vi "LABVIEW_0416043.vi"() -> ()   [LabVIEW 2012]
uses:
  <vilib>/Utility/file.llb/Read From Spreadsheet File (DBL).vi
  <vilib>/Analysis/2dsp.llb/Real FFT.vi
  <vilib>/Analysis/NI_AALPro.lvlib
panel:
  out "Numeric 2":ext
  out "Numeric":ext
  out "FFT {X}":dbl[][](graph)
  out "CSV file path":path
  out "Input1":dbl[](graph)
  # "1. ¶}±ÒÀÉ®×¡AÆ[¹îŠ‹xe®t²§¡C  (ÀÉ¦W:XXX.csv)"
  # "4. HTþsŠ‹xe„vFFT"
  # "3. iQŠ‹xeKNBfßWW"
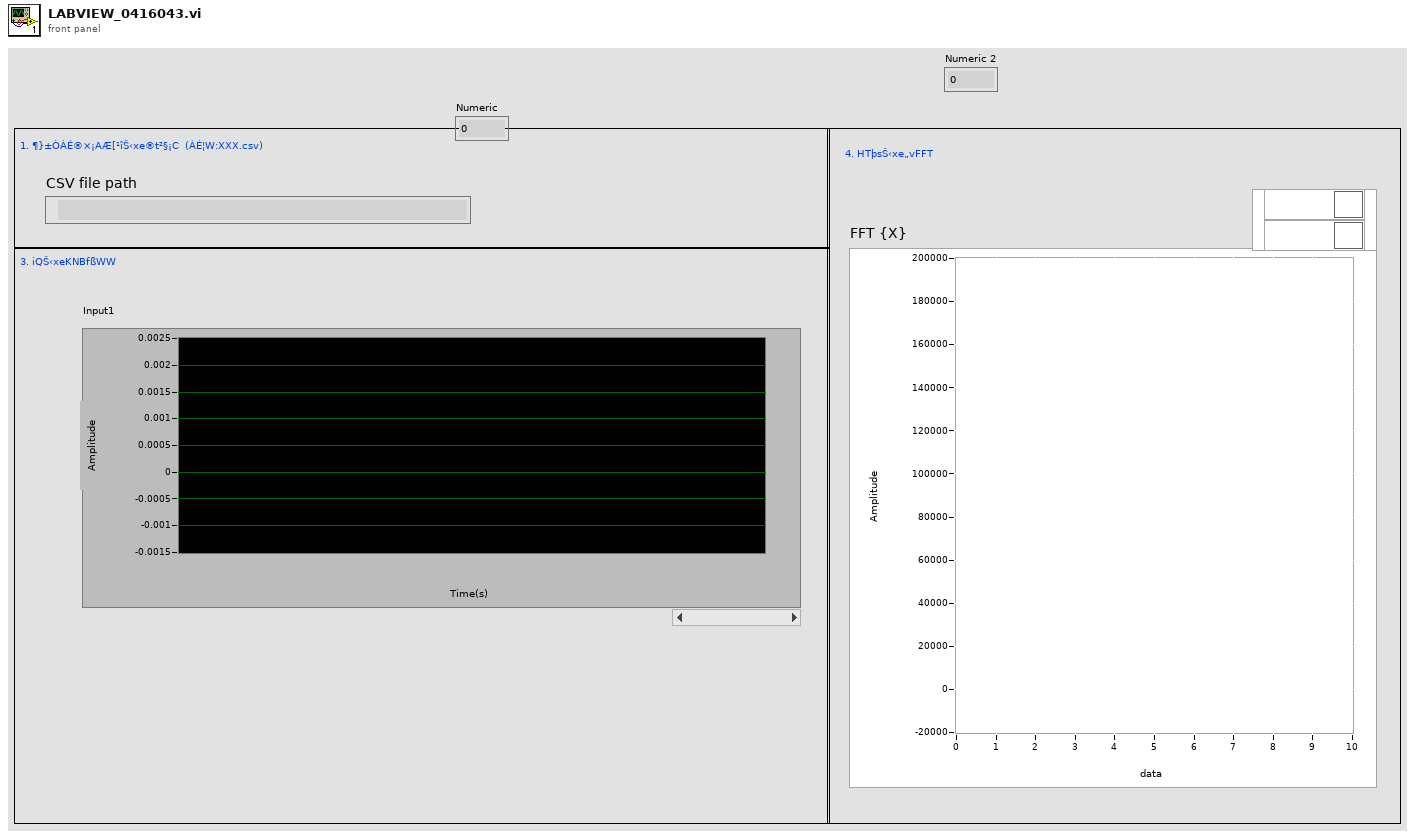
[diagram p1: front panel]
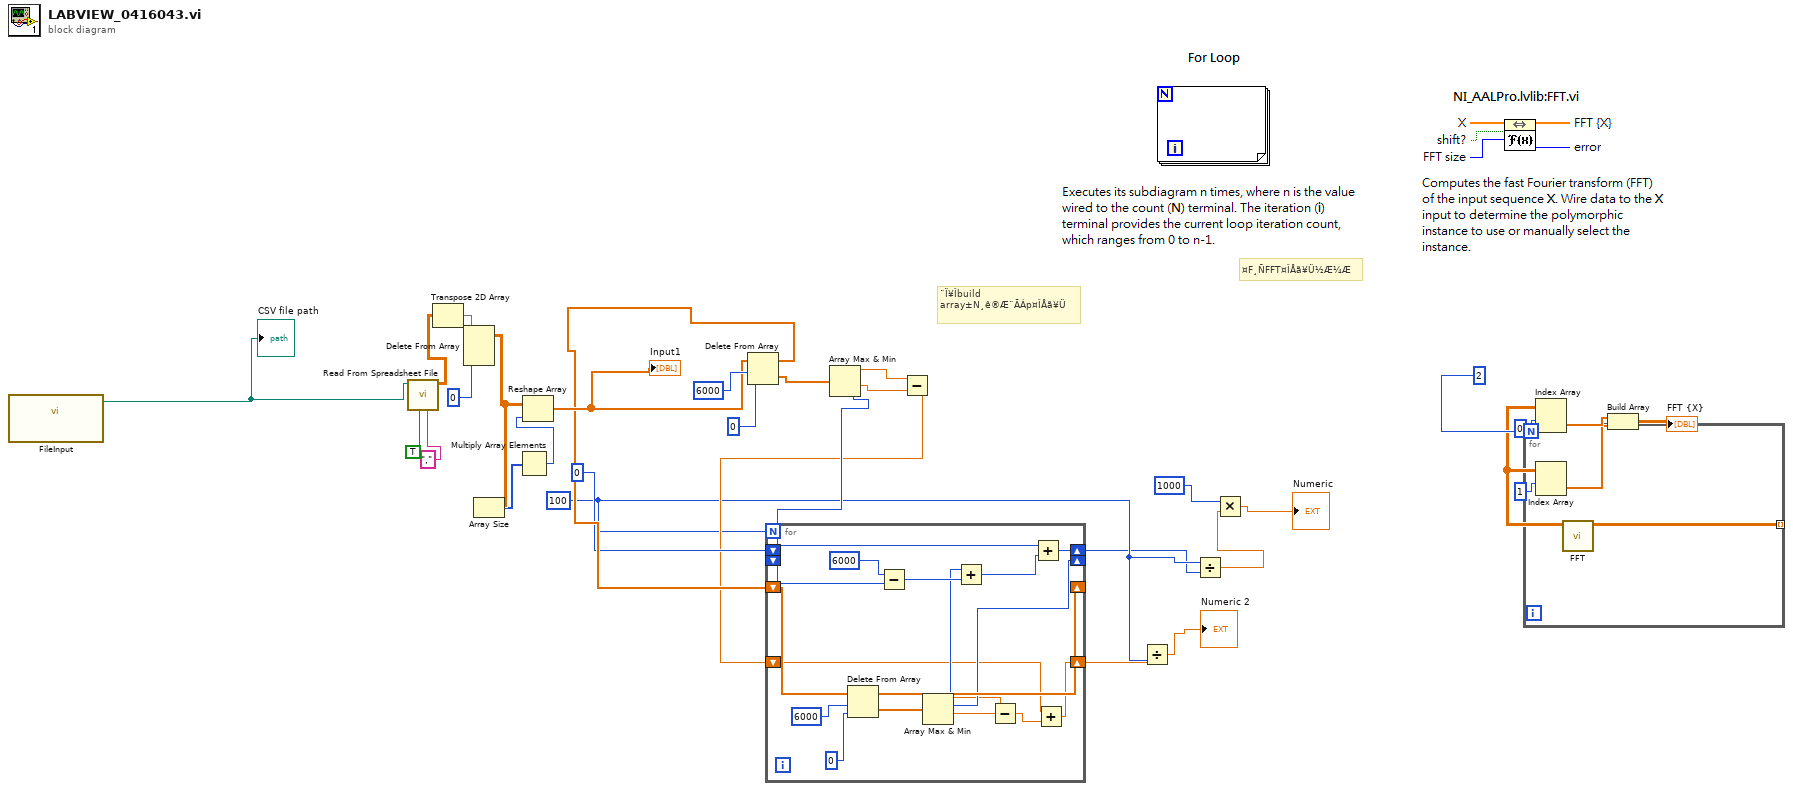
[diagram p0: block diagram]
diagram:
  w5 = 100
  # "了解FFT及顯示複數"
  # "使用build array將資料並聯及顯示"
  n1 = call "FileInput.vi"() -> ("Path"=w27:path)  [unwired: 18 in, 1 out]
  "CSV file path" <- w27
  n2 = call-poly <vilib>:"Read From Spreadsheet File.vi"("delimiter (\\t)"="," ("delimiter (\\t)"), "transpose (no:F)"=TRUE, "file path (dialog if empty)"=w27) -> ("all rows"=w21:dbl[][])  [unwired: 4 in, 4 out]
  n3 = Transpose 2D Array(2D array=w21) -> (transposed array=w20:dbl[][])
  n4 = Delete From Array(array=w20, index (col)=0) -> (array with subset deleted=w24:dbl[][])  [unwired: 2 in, 1 out]
  n5 = Array Size(array=w24) -> (size(s)=w23:i32[])
  n6 = Multiply Array Elements(1:w23) -> (0:w22:i32)
  n7 = Reshape Array(w24, w22) -> (w15:dbl[])
  "Input1" <- w15
  n8 = Delete From Array(array=w15, length=6000, index=0) -> (deleted portion=w14:dbl[], array with subset deleted=w13:dbl[])
  n9 = Array Max & Min(array=w14) -> (max value=w7:dbl, max index (indices)=w12:i32, min value=w10:dbl)  [unwired: 1 out]
  n10 = Subtract(x=w7, y=w10) -> (x-y=w8:dbl)
  n11 = for {
    N: w5 -> [_]
    shift-right: [w46] -> _
    shift-left: w13 -> [w47]
    shift-right: [w39] -> _
    shift-left: w12 -> [w42]
    shift-right: [w45] -> w4
    shift-left: 0 -> [w44]
    shift-right: [w35] -> w9
    shift-left: w8 -> [w34]
    n12 = Delete From Array(array=w47, length=6000, index=0) -> (deleted portion=w48:dbl[], array with subset deleted=w46:dbl[])
    n13 = Subtract(x=6000, y=w42) -> (x-y=w41:i32)
    n14 = Array Max & Min(array=w48) -> (max value=w38:dbl, max index (indices)=w39:i32, min value=w37:dbl)  [unwired: 1 out]
    n15 = Add(x=w39, y=w41) -> (x+y=w40:i32)
    n16 = Subtract(x=w38, y=w37) -> (x-y=w36:dbl)
    n17 = Add(x=w44, y=w40) -> (x+y=w45:i32)
    n18 = Add(x=w34, y=w36) -> (x+y=w35:dbl)
  }
  n19 = Divide(x=w9, y=w5) -> (x/y=→"Numeric 2":dbl)
  n20 = Divide(x=w5, y=w4) -> (x/y=w3:dbl)
  n21 = Multiply(x=1000, y=w3) -> (x*y=→"Numeric":dbl)
  n22 = for {
    N: 2 -> [_]
    tunnel: [w51] -> w18 mode=indexing
    n23 = call-poly <vilib>:"FFT.vi"() -> ("FFT {X}"=w51:cdb[])  [unwired: 10 in, 1 out]
  }
  n24 = Index Array "Index Array"(array=w18, index (row)=0 ("disabled index (col)")) -> (element=w32:cdb[])  [unwired: 1 in]
  n25 = Index Array "Index Array"(array=w18, index (row)=1 ("disabled index (col)")) -> (element=w31:cdb[])  [unwired: 1 in]
  n26 = Build Array "Build Array"(w32, w31) -> (→"FFT {X}":cdb[][])
